vi "Read settings.vi"(8 "error in (no error)":errorcluster, 10 "settings name":string, 11 "Trace in":refnum<class "Trace.lvclass">) -> (0 "error out":errorcluster, 1 "loaded?":bool, 2 "setting name":string, 3 "Trace out":refnum<class "Trace.lvclass">)   [LabVIEW 2012, in "Trace.lvclass"]
doc: "Reads the XML-based settings file and populates the settings cluster accordingly. Settings file name is <component ID>.xml."
uses:
  Trace.lvclass
  <vilib>/Distrio/Murmex/Murmex/Murmex.lvclass
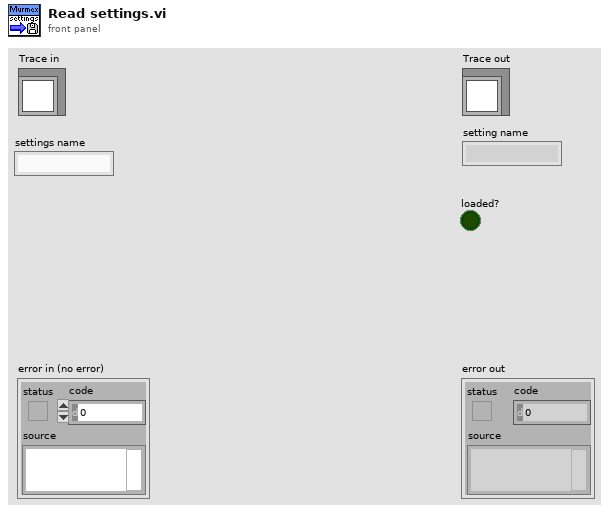
[diagram p1: front panel]
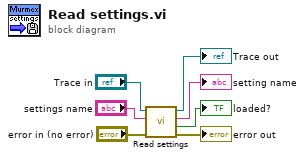
[diagram p0: block diagram]
diagram:
  n1 = call-parent "Read settings.vi"("error in (no error)"="error in (no error)", "settings name"="settings name", "Murmex in"="Trace in") -> ("error out"=→"error out":errorcluster, "loaded?"=→"loaded?":bool, "setting name"=→"setting name":string, "Murmex out"=→"Trace out":refnum<class "Trace.lvclass">)  [unwired: 5 in]
